vi "Start Sync.vi"(8 "error in (no error)":errorcluster, 11 "gRPC Server in":refnum<class "MeasurementPluginService.lvclass">) -> (0 "error out":errorcluster, 3 "gRPC Server out":refnum<class "MeasurementPluginService.lvclass">)   [LabVIEW 2020, in "MeasurementLink Measurement Server.lvlib" / "MeasurementPluginService.lvclass"]
uses:
  MeasurementPluginService.lvclass
  \\10.1.133.57\measurement-services-labview/Source/Measurement Service Template_lv/MeasurementLink Measurement Server Internal/RPC Service/MeasurementService/MeasurementService.lvclass
  MeasurementLink Measurement Server Internal/RPC Service/MeasurementService/MeasurementService.lvclass/MeasurementService.ctl
  MeasurementLink Measurement Server Internal/RPC Messages/ni_measurementlink_measurement_v1_GetMetadataResponse.ctl
  MeasurementLink Measurement Server Internal/RPC Messages/ni_measurementlink_measurement_v1_MeasurementDetails.ctl
  MeasurementLink Measurement Server Internal/RPC Messages/ni_measurementlink_measurement_v1_MeasurementSignature.ctl
  MeasurementLink Measurement Server Internal/RPC Messages/ni_measurementlink_measurement_v1_ConfigurationParameter.ctl
  MeasurementLink Measurement Server Internal/RPC Messages/ni_measurementlink_measurement_v1_ConfigurationParameter_AnnotationsEntry.ctl
  MeasurementLink Measurement Server Internal/RPC Messages/google_protobuf_Any.ctl
  MeasurementLink Measurement Server Internal/RPC Messages/ni_measurementlink_measurement_v1_Output.ctl
  MeasurementLink Measurement Server Internal/RPC Messages/ni_measurementlink_measurement_v1_UserInterfaceDetails.ctl
  MeasurementPluginService.lvclass/MeasurementPluginService.ctl
  MeasurementLink Measurement Server Internal/RPC Service/MeasurementService/MeasurementService.lvclass
  MeasurementLink Measurement Server Internal/MeasurementLink Measurement Server Internal.lvlib
  MeasurementLink Measurement Server.lvlib
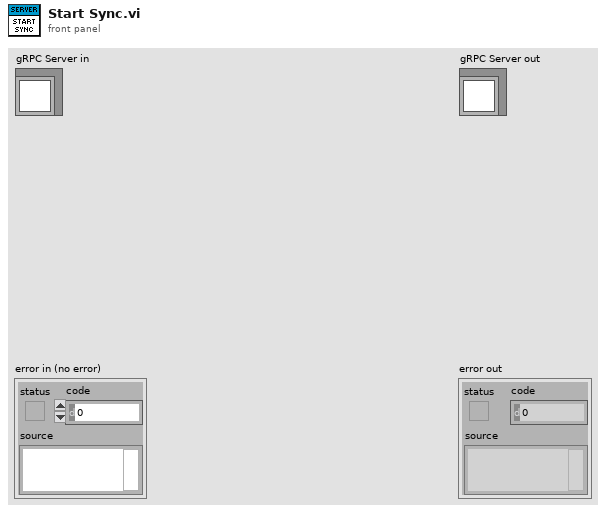
[diagram p1: front panel]
types:
  T1 = typedef "MeasurementLink Measurement Server Internal.lvlib/ni_measurementlink_measurement_v1_MeasurementSignature.ctl" = cluster{"configuration_parameters_message_type":string, "configuration_parameters":T2[], "configuration_defaults":T4, "outputs_message_type":string, "outputs":T5[]}
  T2 = typedef "MeasurementLink Measurement Server Internal.lvlib/ni_measurementlink_measurement_v1_ConfigurationParameter.ctl" = cluster{"field_number":i32, "type":i32, "name":string, "repeated":bool, "annotations":T3[]}
  T3 = typedef "MeasurementLink Measurement Server Internal.lvlib/ni_measurementlink_measurement_v1_ConfigurationParameter_AnnotationsEntry.ctl" = cluster{"key":string, "value":string}
  T4 = typedef "MeasurementLink Measurement Server Internal.lvlib/google_protobuf_Any.ctl" = cluster{"type_url":string, "value":u8[]}
  T5 = typedef "MeasurementLink Measurement Server Internal.lvlib/ni_measurementlink_measurement_v1_Output.ctl" = cluster{"field_number":i32, "type":i32, "name":string, "repeated":bool}
  T6 = typedef "MeasurementLink Measurement Server Internal.lvlib/ni_measurementlink_measurement_v1_GetMetadataResponse.ctl" = cluster{"measurement_details":T7, "measurement_signature":T1, "user_interface_details":T8[]}
  T7 = typedef "MeasurementLink Measurement Server Internal.lvlib/ni_measurementlink_measurement_v1_MeasurementDetails.ctl" = cluster{"display_name":string, "version":string}
  T8 = typedef "MeasurementLink Measurement Server Internal.lvlib/ni_measurementlink_measurement_v1_UserInterfaceDetails.ctl" = cluster{"file_url":string}
  T9 = typedef "MeasurementLink Measurement Server Internal.lvlib/MeasurementService.lvclass/Server Internal UEs.ctl" = cluster{"MeasurementService GetMetadata Internal UE":refnum<user-event>, "MeasurementService Measure Internal UE":refnum<user-event>}
  T10 = typedef "MeasurementLink Measurement Server Internal.lvlib/MeasurementService.lvclass/Server gRPC UEs.ctl" = cluster{"MeasurementService GetMetadata gRPC UE":refnum<user-event>, "MeasurementService Measure gRPC UE":refnum<user-event>}
  T11 = typedef "grpc-lvsupport-release.lvlib/grpcId.ctl" = u64
  T12 = typedef "MeasurementLink Measurement Server.lvlib/MeasurementPluginService.lvclass/Plugin Paths.ctl" = cluster{"Get Measurement Details VI Path":path, "Get Type Specializations VI Path":path, "Get UI Details VI Path":path, "Measurement Logic VI Path":path, "Measurement Configuration CTL Path":path, "Measurement Results CTL Path":path}
  T13 = typedef "grpc-lvsupport-release.lvlib/Any.ctl" = cluster{"Type Url":string, "Bytes":u8[]}
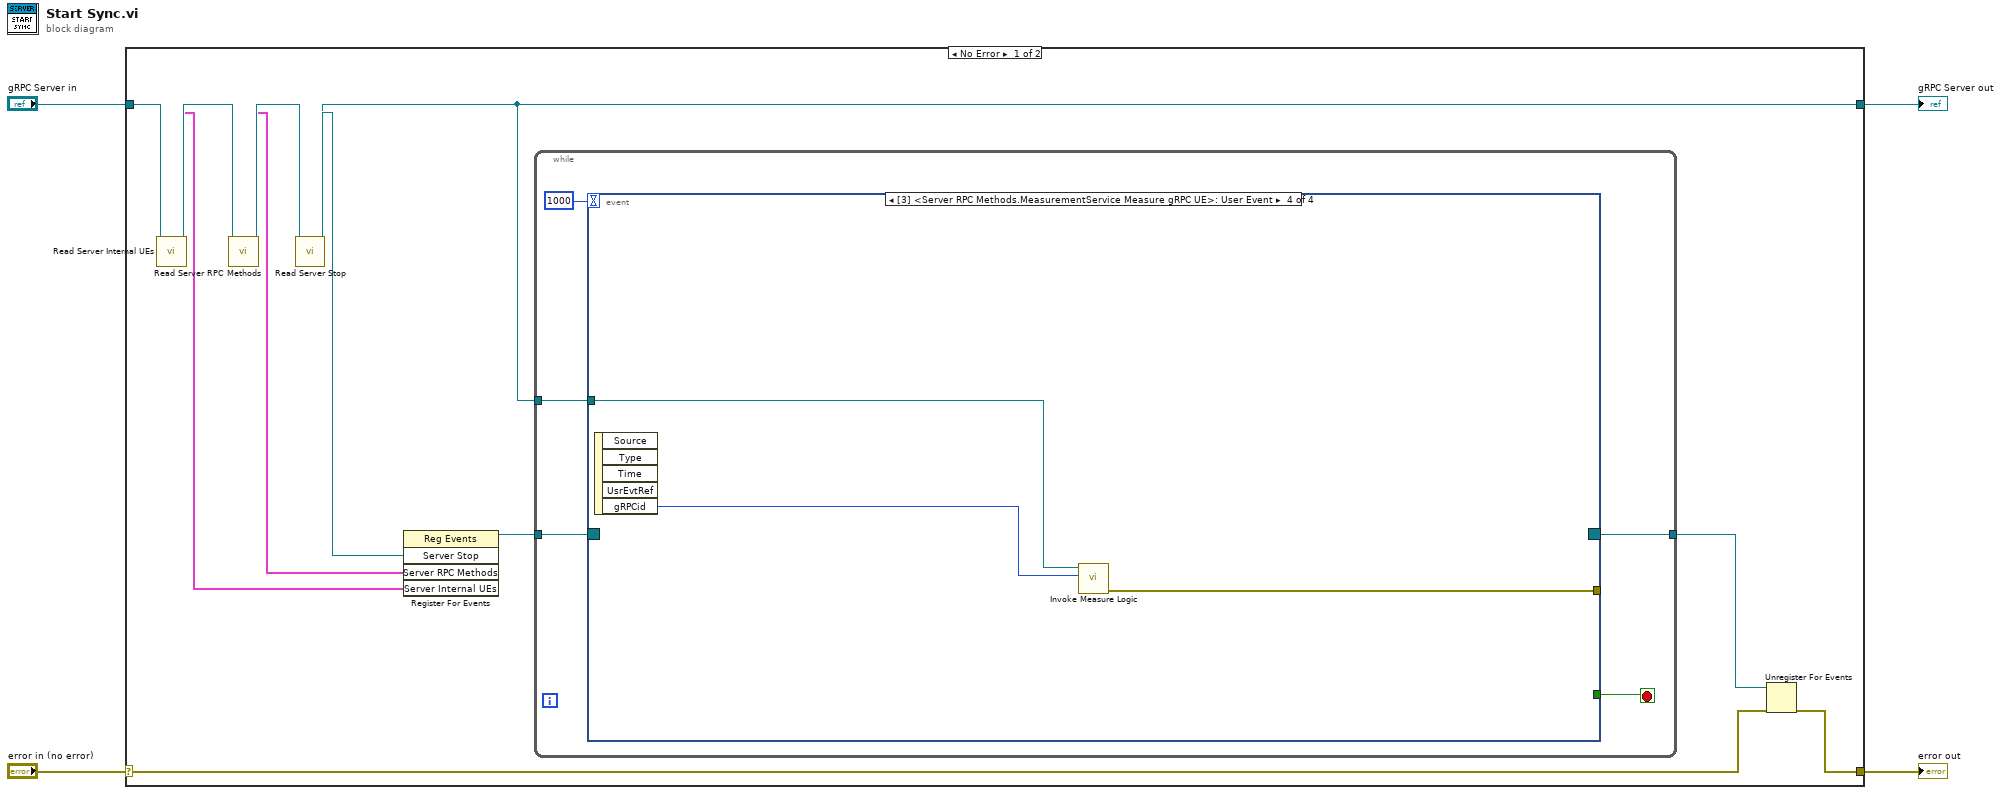
[diagram p0: block diagram]
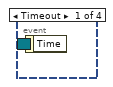
[diagram p2: hidden frame]
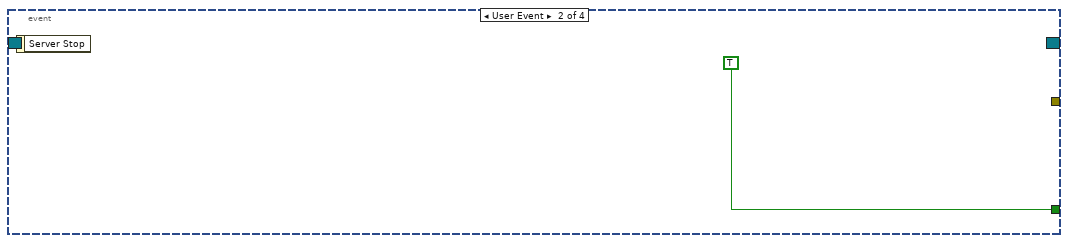
[diagram p3: hidden frame]
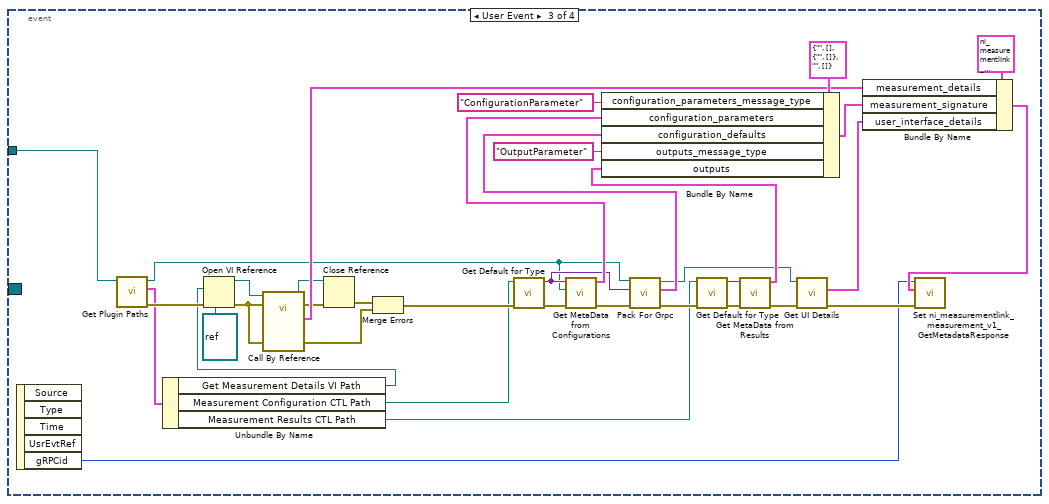
[diagram p4: hidden frame]
diagram:
  n1 = case shown="No Error" "error in (no error)" {
    selector: "error in (no error)" -> [w9 w62]
    tunnel: [w8 w62] -> w3
    tunnel: [w5 w61] -> w1
    tunnel: "gRPC Server in" -> [w15 w61]
    frame No Error {
      n2 = call "Read Server Internal UEs.vi"("SignalGeneratorService in"=w15) -> ("Server Internal UEs"=w13:T9, "SignalGeneratorService out"=w14:refnum<class "MeasurementPluginService.lvclass">)  [unwired: 8 in, 1 out]
      n3 = call "Read Server RPC Methods.vi"("SignalGeneratorService in"=w14) -> ("Server RPC Methods"=w7:T10, "SignalGeneratorService out"=w12:refnum<class "MeasurementPluginService.lvclass">)  [unwired: 8 in, 1 out]
      n4 = call-dynamic "Read Server Stop.vi"("iService in"=w12) -> ("Server Stop"=w6:refnum<user-event>, "iService out"=w5:refnum<class "MeasurementPluginService.lvclass">)  [unwired: 8 in, 1 out]
      n5 = register-events(w6, w7, w13) -> (reference out=w11:refnum<event-registration>)  [unwired: 2 in, 1 out]
      n6 = while {
        tunnel: w11 -> [w20]
        tunnel: [w18] -> w10
        tunnel: w5 -> [w16]
        stop <- w19 stop-if-true
        n7 = event "RPC Methods Event Structure" shown="[3] <Server RPC Methods.MeasurementService Measure gRPC UE>: User Event" {
          selector: w20 -> [_ _ _ _]
          dyn-events: [_ _ _ _] -> w18
          timeout: 1000 -> [_ _ _ _]
          tunnel: [_ TRUE _ _] -> w19
          tunnel: w16 -> [_ _ w29 w60]
          tunnel: [_ _ _ w58] -> _
          event Timeout {
            n8 = event-data() -> ()  [unwired: 1 in, 1 out]
          }
          event User Event {
            n9 = event-data() -> ()  [unwired: 1 in, 1 out]
          }
          event User Event {
            n10 = event-data() -> ("gRPCid"=w35:T11)  [unwired: 1 in, 4 out]
            n11 = call-dynamic "Get Plugin Paths.vi"("MeasurementService in"=w29) -> ("error out"=w28:errorcluster, "Plugin Paths"=w25:T12, "MeasurementService out"=w26:refnum<class "MeasurementPluginService.lvclass">)  [unwired: 8 in]
            n12 = Unbundle By Name(w25) -> ("Get Measurement Details VI Path"=w22:path, "Measurement Configuration CTL Path"=w24:path, "Measurement Results CTL Path"=w23:path)
            n13 = Open VI Reference(type specifier VI Refnum (for type only)=refnum<vi> refnum, vi path=w22, error in (no error)=w28) -> (vi reference=w46:refnum<vi>, error out=w43:errorcluster)  [unwired: 3 in]
            n14 = call-by-ref "?"(reference=w46, error in=w43, "error in"=w43) -> (reference out=w41:refnum<vi>, error out=w40:errorcluster, 0:"error out"=w42:errorcluster, "Measurement Details"=w44:T7)  [unwired: 8 in, 1 out]
            n15 = Close Reference(reference=w41, error in (no error)=w40) -> (error out=w39:errorcluster)
            n16 = Merge Errors(w39, w42) -> (w38:errorcluster)
            n17 = call "Get Default for Type.vi"("error in (no error)"=w38, "Path of Type"=w24) -> ("error out"=w52:errorcluster, "Default for Type"=w33:variant)  [unwired: 8 in]
            n18 = call "Get MetaData from Configurations.vi"("error in"=w52, "Measurement"=w26, "Configuration Cluster"=w33) -> ("error out"=w34:errorcluster, "configuration_parameters"=w57:T2[])  [unwired: 7 in]
            n19 = call-dynamic "Pack For Grpc.vi"("error in (no error)"=w34, "Data Value"=w33, "gRPC Server in"=w26) -> ("error out"=w31:errorcluster, "Any"=w32:T13, "gRPC Server out"=w27:refnum<class "MeasurementPluginService.lvclass">)  [unwired: 6 in]
            n20 = call "Get Default for Type.vi"("error in (no error)"=w31, "Path of Type"=w23) -> ("error out"=w36:errorcluster, "Default for Type"=w37:variant)  [unwired: 8 in]
            n21 = call "Get MetaData from Results.vi"("error in"=w36, "Configuration Cluster"=w37) -> ("error out"=w53:errorcluster, "outputs"=w56:T5[])  [unwired: 8 in]
            n22 = Bundle By Name(cluster=T1 {"configuration_parameters_message_type"="", "configuration_parameters"=[], "configuration_defaults"={"type_url"="", "value"=[]}, "outputs_message_type"="", "outputs"=[]} ("ni_measurements_v1_MeasurementSignature"), "configuration_parameters_message_type"="ConfigurationParameter" ("configuration_parameters_messagetype"), "configuration_parameters"=w57, "configuration_defaults"=w32, "outputs_message_type"="OutputParameter" ("configuration_parameters_messagetype"), "outputs"=w56) -> (w48:T1)
            n23 = call-dynamic "Get UI Details.vi"("error in"=w53, "gRPC Server in"=w27) -> ("error out"=w50:errorcluster, "user_interface_details"=w30:T8[])  [unwired: 7 in, 1 out]
            n24 = Bundle By Name(cluster=T6 {"measurement_details"={"display_name"="", "version"=""}, "measurement_signature"={"configuration_parameters_message_type"="", "configuration_parameters"=[], "configuration_defaults"={"type_url"="", "value"=[]}, "outputs_message_type"="", "outputs"=[]}, "user_interface_details"=[]} ("package_templatemessage"), "measurement_details"=w44, "measurement_signature"=w48, "user_interface_details"=w30) -> (w49:T6)
            n25 = call "Set ni_measurementlink_measurement_v1_GetMetadataResponse.vi"("error in (no error)"=w50, "package_templatemessage"=w49, "gRPCid"=w35) -> ()  [unwired: 8 in, 1 out]
          }
          event User Event {
            n26 = event-data() -> ("gRPCid"=w59:T11)  [unwired: 1 in, 4 out]
            n27 = call "Invoke Measure Logic.vi"("gRPCid in"=w59, "gRPC Server in"=w60) -> ("error out"=w58:errorcluster)  [unwired: 9 in]
          }
        }
      }
      n28 = Unregister For Events(event registration refnum=w10, error in=w9) -> (error out=w8:errorcluster)
    }
    frame Error {
    }
  }
  "error out" <- w3
  "gRPC Server out" <- w1
